vi "edge_scan_z.vi"(7 "error in (no error)":errorcluster, 9 "z_scan_params":T2={"-offset"=-200.0, "+offset"=200.0, "speed"=0.5, "threshold"=4.0, "y-offset"=50.0}, 10 "refs":T4) -> (0 "error out":errorcluster, 1 "graph":cluster{sgl[], dbl[]}, 2 "z_out":sgl, 3 "refs out":T4)   [LabVIEW 2018]
uses:
  C:/Program Files/National Instruments/LabVIEW 2018/instr.lib/IDS/ueye.NET/uEyeDotNet.dll
  <userlib>/PDamp/PDref.ctl
  <userlib>/stepper/velocity settings.ctl
  <userlib>/PDamp/channel.ctl
panel:
  in  "velocity parameters in":T1={"pfMinVel"=0.0, "pfAccn"=4.0, "pfMaxVel"=4.0}
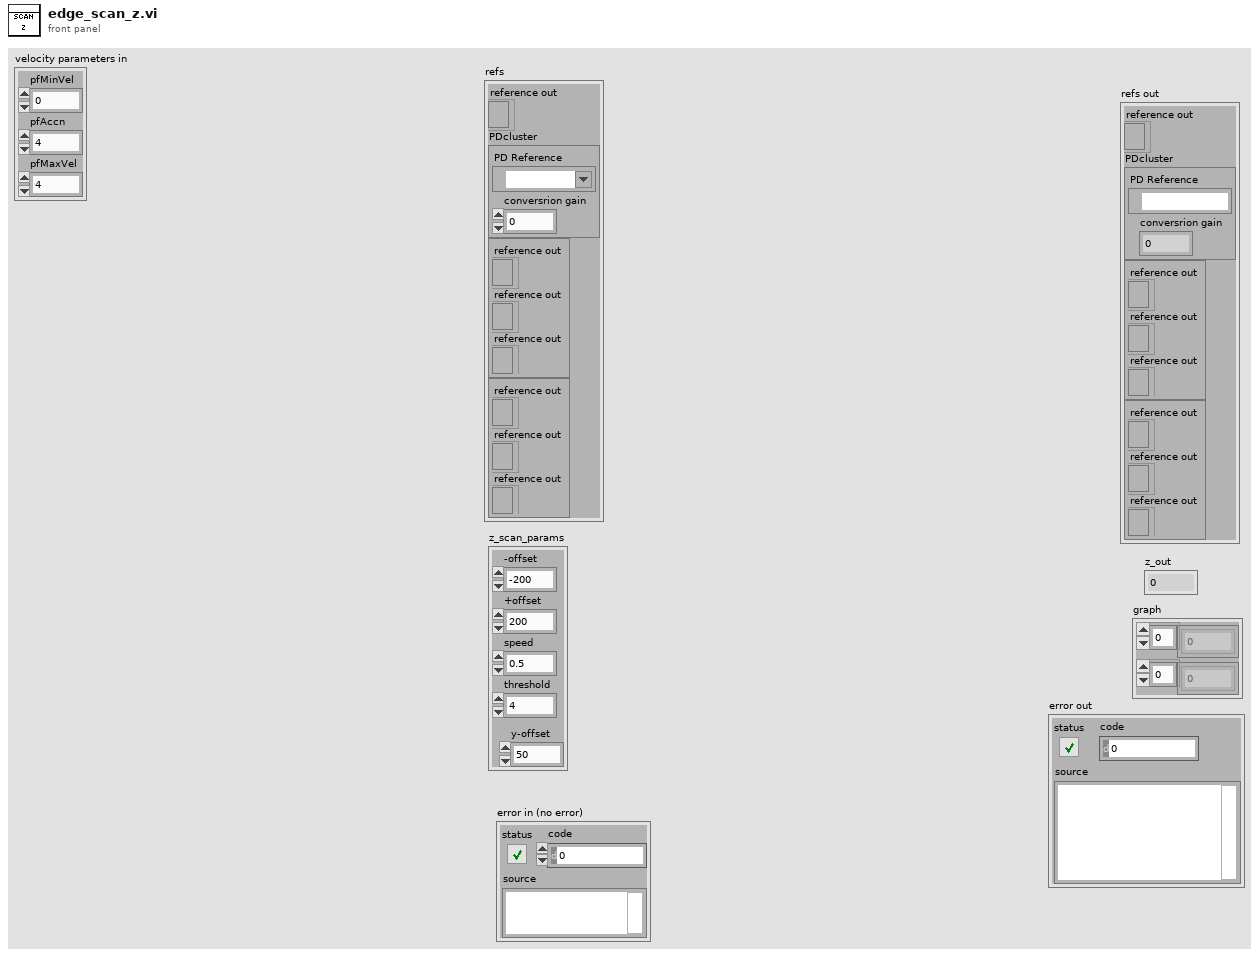
[diagram p1: front panel]
types:
  T1 = typedef "velocity settings.ctl" = cluster{"pfMinVel":sgl, "pfAccn":sgl, "pfMaxVel":sgl}
  T2 = cluster{"-offset":sgl, "+offset":sgl, "speed":sgl, "threshold":dbl, "y-offset":dbl}
  T3 = typedef "PDref.ctl" = cluster{"PD Reference":refnum<visa-resource-name>, "conversrion gain":dbl}
  T4 = cluster{"reference out":refnum<k24>, "PDcluster":T3, cluster{"reference out":refnum<k7>, "reference out":refnum<k7>, "reference out":refnum<k7>}, cluster{"reference out":refnum<k7>, "reference out":refnum<k7>, "reference out":refnum<k7>}}
  T5 = cluster{"reference out":refnum<k7>, "reference out":refnum<k7>, "reference out":refnum<k7>}
  T6 = typedef "channel.ctl" = enum16{"ch1", "ch2", "ch3", "ch4"}
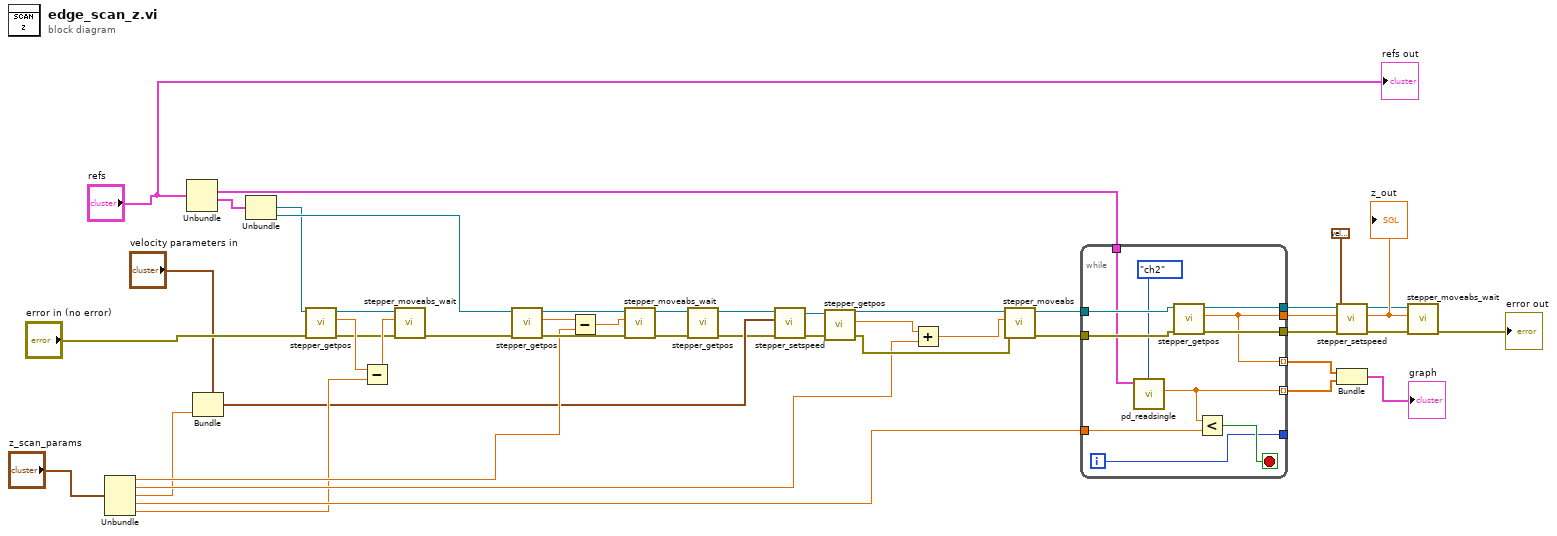
[diagram p0: block diagram]
diagram:
  n1 = Unbundle("z_scan_params") -> ("-offset"=w14:sgl, "+offset"=w13:sgl, "speed"=w12:sgl, "threshold"=w11:dbl, "y-offset"=w10:dbl)
  n2 = Unbundle("refs") -> ("PDcluster"=w31:T3, w45:T5)  [unwired: 2 out]
  n3 = Bundle(cluster="velocity parameters in", "pfMaxVel"=w12) -> (w6:T1)  [unwired: 2 in]
  n4 = Unbundle(w45) -> ("reference out"=w18:refnum<k7>, "reference out"=w44:refnum<k7>)  [unwired: 1 out]
  n5 = call <userlib>:"stepper_getpos.vi"("error in (no error)"="error in (no error)", "reference"=w18) -> ("error out"=w16:errorcluster, "pfPosition[µm]"=w17:sgl, "reference out"=w19:refnum<k7>)  [unwired: 7 in]
  n6 = Subtract(x=w17, y=w10) -> (x-y=w21:dbl)
  n7 = call <userlib>:"stepper_moveabs_wait.vi"("error in (no error)"=w16, "fAbsPos[µm]"=w21, "reference"=w19) -> ("error out"=w42:errorcluster)  [unwired: 7 in, 1 out]
  n8 = call <userlib>:"stepper_getpos.vi"("error in (no error)"=w42, "reference"=w44) -> ("error out"=w40:errorcluster, "pfPosition[µm]"=w41:sgl, "reference out"=w43:refnum<k7>)  [unwired: 7 in]
  n9 = Subtract(x=w41, y=w14) -> (x-y=w1:sgl)
  n10 = call <userlib>:"stepper_moveabs_wait.vi"("error in (no error)"=w40, "fAbsPos[µm]"=w1, "reference"=w43) -> ("error out"=w4:errorcluster, "reference out"=w5:refnum<k7>)  [unwired: 7 in]
  n11 = call <userlib>:"stepper_getpos.vi"("error in (no error)"=w4, "reference"=w5) -> ("error out"=w3:errorcluster, "reference out"=w2:refnum<k7>)  [unwired: 7 in, 1 out]
  n12 = call <userlib>:"stepper_setspeed.vi"("error in (no error)"=w3, "velocity parameters in"=w6, "reference"=w2) -> ("error out"=w39:errorcluster, "reference out"=w38:refnum<k7>)  [unwired: 6 in, 1 out]
  n13 = call <userlib>:"stepper_getpos.vi"("error in (no error)"=w39, "reference"=w38) -> ("error out"=w33:errorcluster, "pfPosition[µm]"=w37:sgl, "reference out"=w36:refnum<k7>)  [unwired: 7 in]
  n14 = Add(x=w37, y=w13) -> (x+y=w35:sgl)
  n15 = call <userlib>:"stepper_moveabs.vi"("error in (no error)"=w33, "fAbsPos[µm]"=w35, "reference"=w36) -> ("error out"=w32:errorcluster, "reference out"=w34:refnum<k7>)  [unwired: 7 in]
  n16 = while {
    tunnel: w34 -> [w55]
    tunnel: w32 -> [w56]
    tunnel: w31 -> [w54]
    tunnel: [w53] -> w28 mode=indexing
    tunnel: [w48] -> w30
    tunnel: w11 -> [w52]
    tunnel: [w50] -> w24
    tunnel: [w49] -> w26
    tunnel: [w48] -> w29 mode=indexing
    tunnel: [w47] -> _
    i -> [w47]
    stop <- w51 stop-if-true
    n17 = call <userlib>:"pd_readsingle.vi"("PDcluster in"=w54, "channel"=channel."ch2") -> ("photocurrent"=w53:dbl)  [unwired: 6 in, 2 out]
    n18 = call <userlib>:"stepper_getpos.vi"("error in (no error)"=w56, "reference"=w55) -> ("error out"=w49:errorcluster, "pfPosition[µm]"=w48:sgl, "reference out"=w50:refnum<k7>)  [unwired: 7 in]
    n19 = Less?(x=w53, y=w52) -> (x < y?=w51:bool)
  }
  "z_out" <- w30
  n20 = call <userlib>:"stepper_setspeed.vi"("error in (no error)"=w26, "velocity parameters in"=T1 {"pfMinVel"=0.0, "pfAccn"=4.0, "pfMaxVel"=4.0}, "reference"=w24) -> ("error out"=w25:errorcluster, "reference out"=w23:refnum<k7>)  [unwired: 6 in, 1 out]
  n21 = Bundle(w29, w28) -> (→"graph":cluster{sgl[], dbl[]})  [unwired: 1 in]
  n22 = call <userlib>:"stepper_moveabs_wait.vi"("error in (no error)"=w25, "fAbsPos[µm]"=w30, "reference"=w23) -> ("error out"=→"error out":errorcluster)  [unwired: 7 in, 1 out]
  "refs out" <- "refs"
